vi "checkStatus.vi"(8 "error in (no error)":errorcluster, 10 "stop":bool, 11 "NetworkPixelfly in":refnum<class "NetworkPixelfly.lvclass">) -> (0 "error out":errorcluster, 2 "stopped?":bool, 3 "NetworkPixelfly out":refnum<class "NetworkPixelfly.lvclass">)   [LabVIEW 2009, in "Hardware.lvlib" / "HWControllers.lvlib" / "NetworkPixelfly.lvclass"]
uses:
  NetworkPixelfly.lvclass
  NetworkCamera.lvclass
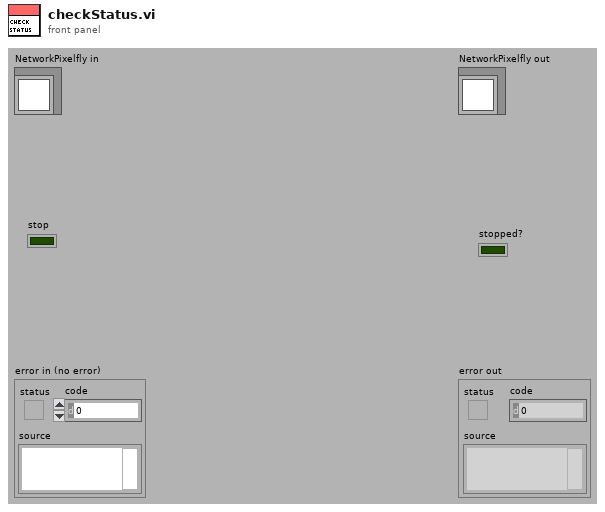
[diagram p1: front panel]
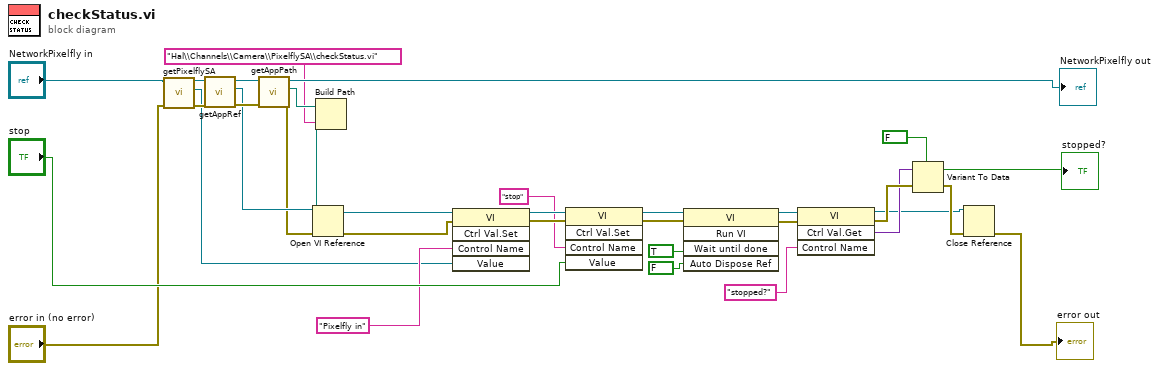
[diagram p0: block diagram]
diagram:
  n1 = call "getPixelflySA.vi"("error in (no error)"="error in (no error)", "NetworkCamera in"="NetworkPixelfly in") -> ("error out"=w4:errorcluster, "PixelflySA.lvclass"=w3:refnum<class "PixelflySA.lvclass">, "NetworkCamera out"=w5:refnum<class "NetworkPixelfly.lvclass">)  [unwired: 7 in]
  n2 = call "getAppRef.vi"("error in (no error)"=w4, "NetworkCamera in"=w5) -> ("error out"=w29:errorcluster, "appRef"=w26:refnum<vi>, "NetworkCamera out"=w30:refnum<class "NetworkPixelfly.lvclass">)  [unwired: 7 in]
  n3 = call "getAppPath.vi"("error in (no error)"=w29, "NetworkCamera in"=w30) -> ("error out"=w24:errorcluster, "appPath"=w28:path, "NetworkCamera out"=→"NetworkPixelfly out":refnum<class "NetworkPixelfly.lvclass">)  [unwired: 7 in]
  n4 = Build Path(base path=w28, name or relative path="Hal\\Channels\\Camera\\PixelflySA\\checkStatus.vi") -> (appended path=w25:path)
  n5 = Open VI Reference(application reference (local)=w26, vi path=w25, error in (no error)=w24) -> (vi reference=w7:refnum<vi>, error out=w6:errorcluster)  [unwired: 3 in]
  n6 = invoke class="VI" method="Ctrl Val.Set"(reference=w7, error in=w6, "Control Name"="Pixelfly in", "Value"=w3) -> (reference out=w23:refnum<vi>, error out=w22:errorcluster)  [unwired: 1 in, 3 out]
  n7 = invoke class="VI" method="Ctrl Val.Set"(reference=w23, error in=w22, "Control Name"="stop", "Value"="stop") -> (reference out=w19:refnum<vi>, error out=w20:errorcluster)  [unwired: 1 in, 3 out]
  n8 = invoke class="VI" method="Run VI"(reference=w19, error in=w20, "Wait until done"=TRUE ("Wait Until Done"), "Auto Dispose Ref"=FALSE ("Auto Dispose Reference")) -> (reference out=w15:refnum<vi>, error out=w16:errorcluster)  [unwired: 1 in, 3 out]
  n9 = invoke class="VI" method="Ctrl Val.Get"(reference=w15, error in=w16, "Control Name"="stopped?") -> (reference out=w10:refnum<vi>, error out=w13:errorcluster, "Get Control Value Variant"=w12:variant)  [unwired: 1 in, 1 out]
  n10 = Variant To Data(error in=w13, Variant=w12, type=FALSE) -> (error out=w11:errorcluster, data=→"stopped?":bool)
  n11 = Close Reference(reference=w10, error in (no error)=w11) -> (error out=→"error out":errorcluster)
